vi "closeEvent.vi"(8 "error in (no error)":errorcluster, 11 "PixelflySettings in":refnum<class "PixelflySettings.lvclass">) -> (0 "error out":errorcluster, 3 "PixelflySettings out":refnum<class "PixelflySettings.lvclass">)   [LabVIEW 2011, in "Tools.lvlib" / "Settings.lvlib" / "PixelflySettings.lvclass"]
uses:
  PixelflySettings.lvclass
  PixelflySettings.lvclass/PixelflySettings.ctl
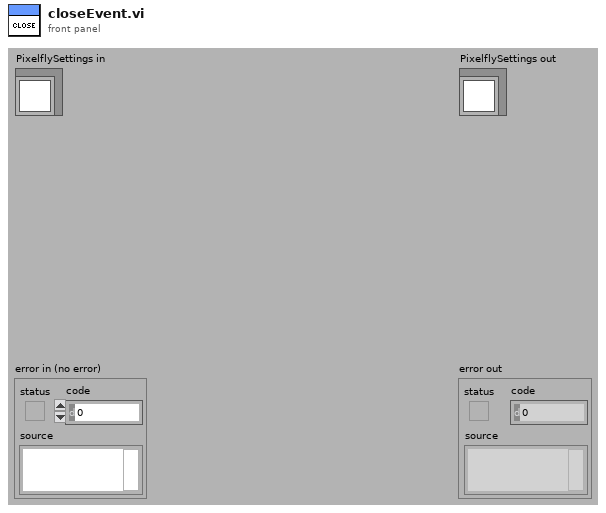
[diagram p1: front panel]
types:
  T1 = enum32{"Invalid", "Standard", "Closed", "Hidden", "Minimized", "Maximized"}
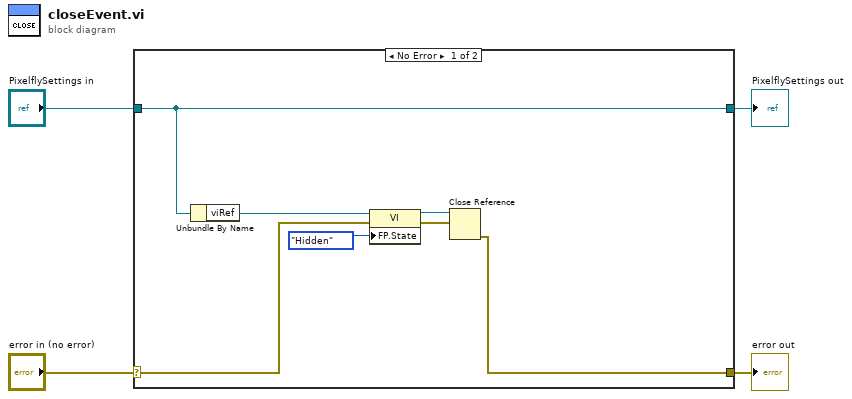
[diagram p0: block diagram]
diagram:
  n1 = case shown="No Error" "error in (no error)" {
    selector: "error in (no error)" -> [w8 w13]
    tunnel: [w7 w13] -> w3
    tunnel: [w6 w12] -> w1
    tunnel: "PixelflySettings in" -> [w6 w12]
    frame No Error {
      n2 = Unbundle By Name(w6) -> ("viRef"=w5:refnum<vi>)
      n3 = property class="VI"(reference=w5, error in=w8, "FP.State"=T1."Hidden" ("Front Panel Window:State")) -> (reference out=w9:refnum<vi>, error out=w10:errorcluster)
      n4 = Close Reference(reference=w9, error in (no error)=w10) -> (error out=w7:errorcluster)
    }
    frame Error {
    }
  }
  "error out" <- w3
  "PixelflySettings out" <- w1
